vi "Append Block.vi"(10 "block in":u8[](array[numeric]) format="%02x", 11 "Hash Function in":refnum<class "NI_SHA-512.lvclass">) -> (3 "Hash Function out":refnum<class "NI_SHA-512.lvclass">)   [LabVIEW 2020, in "NI_SHA-512.lvclass"]
uses:
  <vilib>/security/Message Digest/SHA-2/SHA-512/NI_SHA-512.lvclass
  <vilib>/security/Message Digest/SHA-2/SHA-512/NI_SHA-512.lvclass/NI_SHA-512.ctl
  <vilib>/Bit Manipulation/wrappers/Network-Order Bytes To Words/Network-Order Bytes To Words U64.vi
  <vilib>/Bit Manipulation/NI_Bit Manipulation.lvlib
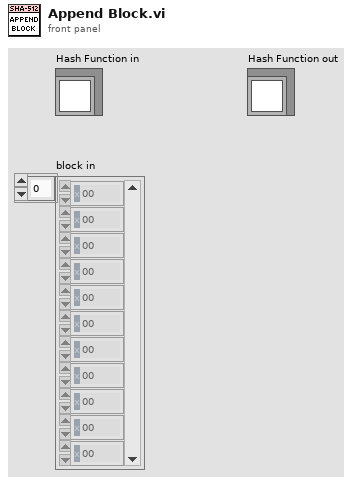
[diagram p1: front panel]
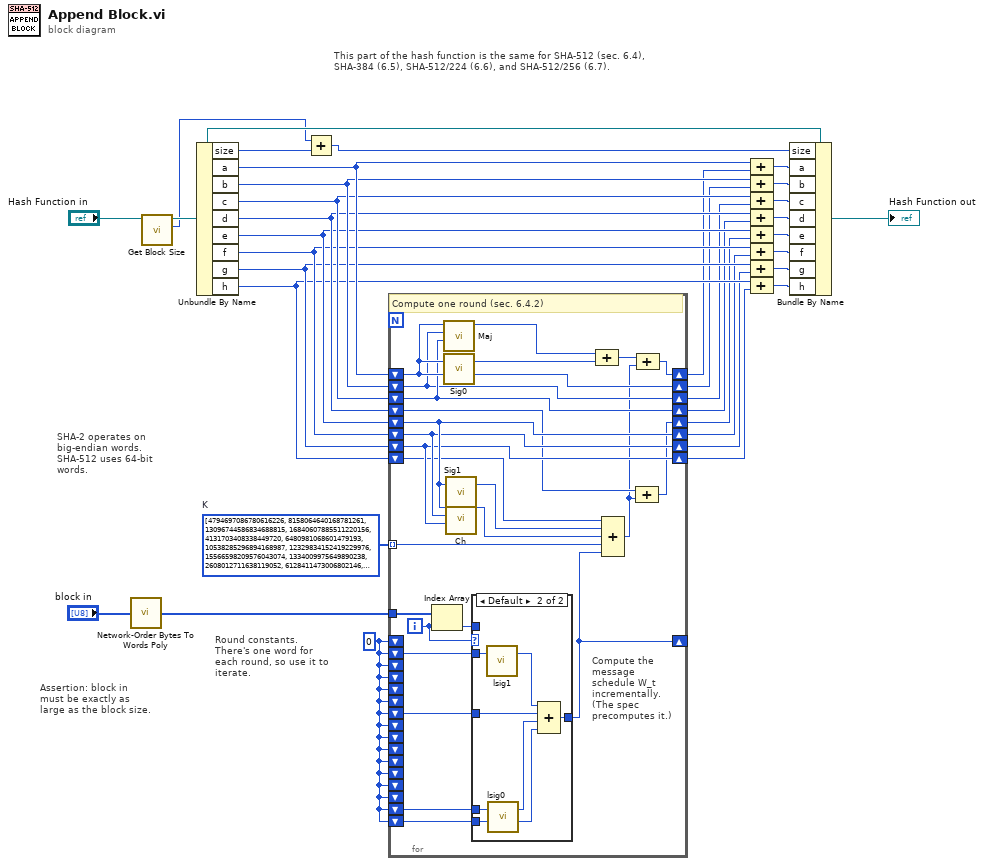
[diagram p0: block diagram]
diagram:
  w1 = u64 0 ("Numeric")
  w10 = u64[] [4794697086780616226, 8158064640168781261, 13096744586834688815, 16840607885511220156, 4131703408338449720, 6480981068601479193, 10538285296894168987, 12329834152419229976, 15566598209576043074, 1334009975649890238, 2608012711638119052, 6128411473006802146, 8268148722764581231, 9286055187155687089, 11230858885718282805, 13951009754708518548, 16472876342353939154, 17275323862435702243, 1135362057144423861, 2597628984639134821, 3308224258029322869, 5365058923640841347, 6679025012923562964, 8573033837759648693, 10970295158949994411, 12119686244451234320, 12683024718118986047, 13788192230050041572, 14330467153632333762, 15395433587784984357, 489312712824947311, 1452737877330783856, 2861767655752347644, 3322285676063803686, 5560940570517711597, 5996557281743188959, 7280758554555802590, 8532644243296465576, 9350256976987008742, 10552545826968843579, 11727347734174303076, 12113106623233404929, 14000437183269869457, 14369950271660146224, 15101387698204529176, 15463397548674623760, 17586052441742319658, 1182934255886127544, 1847814050463011016, 2177327727835720531, 2830643537854262169, 3796741975233480872, 4115178125766777443, 5681478168544905931, 6601373596472566643, 7507060721942968483, 8399075790359081724, 8693463985226723168, 9568029438360202098, 10144078919501101548, 10430055236837252648, 11840083180663258601, 13761210420658862357, 14299343276471374635, 14566680578165727644, 15097957966210449927, 16922976911328602910, 17689382322260857208, 500013540394364858, 748580250866718886, 1242879168328830382, 1977374033974150939, 2944078676154940804, 3659926193048069267, 4368137639120453308, 4836135668995329356, 5532061633213252278, 6448918945643986474, 6902733635092675308, 7801388544844847127]  # K
  # "Round constants. There's one word for each round, so use it to iterate."
  # "This part of the hash function is the same for SHA-512 (sec. 6.4), SHA-384 (6.5), SHA-512/224 (6.6), and SHA-512/256 (6.7)."
  # "Assertion: block in must be exactly as large as the block size."
  # "SHA-2 operates on big-endian words. SHA-512 uses 64-bit words."
  n1 = call-poly <vilib>:"Network-Order Bytes To Words Poly.vi"("bytes in"="block in") -> ("words out"=w32:u64[])
  n2 = call <vilib>:"Get Block Size.vi"("Hash Function in"="Hash Function in") -> ("block size (bytes)"=w29:i32, "Hash Function out"=w30:refnum<class "NI_SHA-512.lvclass">)  [unwired: 9 in]
  n3 = Unbundle By Name(w30) -> ("size"=w28:u64, "a"=w18:u64, "b"=w17:u64, "c"=w16:u64, "d"=w15:u64, "e"=w14:u64, "f"=w13:u64, "g"=w12:u64, "h"=w11:u64)
  n4 = Add(x=w29, y=w28) -> (x+y=w27:u64)
  n5 = for {
    shift-right: [w43] -> w9
    shift-left: w18 -> [w50]
    shift-right: [w50] -> w8
    shift-left: w17 -> [w48]
    shift-right: [w48] -> w7
    shift-left: w16 -> [w49]
    shift-right: [w49] -> w6
    shift-left: w15 -> [w52]
    shift-right: [w51] -> w5
    shift-left: w14 -> [w59]
    shift-right: [w59] -> w4
    shift-left: w13 -> [w58]
    shift-right: [w58] -> w3
    shift-left: w12 -> [w57]
    shift-right: [w57] -> w2
    shift-left: w11 -> [w56]
    tunnel: w10 -> [w53] mode=indexing
    tunnel: w32 -> [w42]
    shift-right: [w35] -> _
    shift-left: w1 -> [_]
    shift-left: w1 -> [w39]
    shift-left: w1 -> [_]
    shift-left: w1 -> [_]
    shift-left: w1 -> [_]
    shift-left: w1 -> [_]
    shift-left: w1 -> [w38]
    shift-left: w1 -> [_]
    shift-left: w1 -> [_]
    shift-left: w1 -> [_]
    shift-left: w1 -> [_]
    shift-left: w1 -> [_]
    shift-left: w1 -> [_]
    shift-left: w1 -> [_]
    shift-left: w1 -> [w37]
    shift-left: w1 -> [w36]
    i -> [w41]
    # "Compute the message schedule W_t incrementally. (The spec precomputes it.)"
    # "Compute one round (sec. 6.4.2)"
    n6 = Index Array(array=w42, index=w41) -> (element=w40:u64)
    n7 = call <vilib>:"Maj.vi"("z"=w49, "y"=w48, "x"=w50) -> ("Maj"=w47:u64)  [unwired: 8 in]
    n8 = call <vilib>:"Sig0.vi"("x"=w50) -> ("Sig0"=w46:u64)  [unwired: 2 in]
    n9 = call <vilib>:"Sig1.vi"("x"=w59) -> ("Sig1"=w55:u64)  [unwired: 2 in]
    n10 = call <vilib>:"Ch.vi"("z"=w57, "y"=w58, "x"=w59) -> ("Ch"=w54:u64)  [unwired: 8 in]
    n11 = case shown="Default" w41 {
      tunnel: w39 -> [_ w67]
      tunnel: w38 -> [_ w65]
      tunnel: w37 -> [_ w64]
      tunnel: w36 -> [_ w62]
      tunnel: [w60 w61] -> w35
      tunnel: w40 -> [w60 _]
      frame 0..15 {
      }
      frame Default {
        n12 = call <vilib>:"lsig1.vi"("x"=w67) -> ("lsig1"=w66:u64)  [unwired: 2 in]
        n13 = call <vilib>:"lsig0.vi"("x"=w64) -> ("lsig0"=w63:u64)  [unwired: 2 in]
        n14 = Compound Arithmetic op=ADD(w66, w65, w63, w62) -> (w61:u64)
      }
    }
    n15 = Compound Arithmetic op=ADD(w47, w46) -> (w45:u64)
    n16 = Compound Arithmetic op=ADD(w56, w55, w54, w53, w35) -> (w44:u64)
    n17 = Compound Arithmetic op=ADD(w52, w44) -> (w51:u64)
    n18 = Compound Arithmetic op=ADD(w45, w44) -> (w43:u64)
  }
  n19 = Compound Arithmetic op=ADD(w18, w9) -> (w26:u64)
  n20 = Compound Arithmetic op=ADD(w17, w8) -> (w25:u64)
  n21 = Compound Arithmetic op=ADD(w16, w7) -> (w24:u64)
  n22 = Compound Arithmetic op=ADD(w15, w6) -> (w23:u64)
  n23 = Compound Arithmetic op=ADD(w14, w5) -> (w22:u64)
  n24 = Compound Arithmetic op=ADD(w13, w4) -> (w21:u64)
  n25 = Compound Arithmetic op=ADD(w12, w3) -> (w20:u64)
  n26 = Compound Arithmetic op=ADD(w11, w2) -> (w19:u64)
  n27 = Bundle By Name(cluster=w30, "size"=w27, "a"=w26, "b"=w25, "c"=w24, "d"=w23, "e"=w22, "f"=w21, "g"=w20, "h"=w19) -> (→"Hash Function out":refnum<class "NI_SHA-512.lvclass">)
